vi "DT_Triangle Manager_Get Local Point Index.vi"(9 "global idx":i32, 10 "triangle":i32, 11 "Triangles":i32[][](array[numeric])) -> (2 "local idx":i32)   [LabVIEW 2017, in "NI_AAL_Geometry.lvlib"]
uses:
  <vilib>/Analysis/NI_AAL_Geometry.lvlib
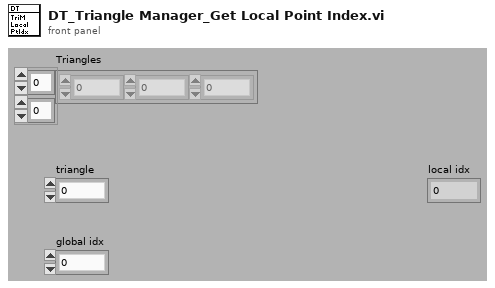
[diagram p1: front panel]
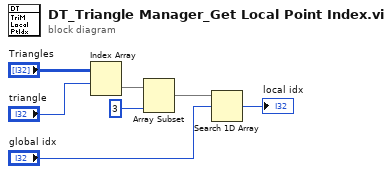
[diagram p0: block diagram]
diagram:
  n1 = Index Array(array="Triangles", index (row)="triangle") -> (element=w5:i32[])  [unwired: 1 in]
  n2 = Array Subset(array=w5, length=3) -> (w6:i32[])  [unwired: 1 in]
  n3 = Search 1D Array(1D array=w6, element="global idx") -> (index of element=→"local idx":i32)  [unwired: 1 out]
